vi "Build CHM.vi"() -> ()   [LabVIEW 2015]
uses:
  <vilib>/Utility/config.llb/Read Key (String).vi
  <vilib>/Utility/config.llb/Read Key (Path).vi
  Classes/CHM Generator/CHM Generator.lvclass
  <vilib>/Utility/config.llb/NI_LVConfig.lvlib
panel:
  out "standard output":string
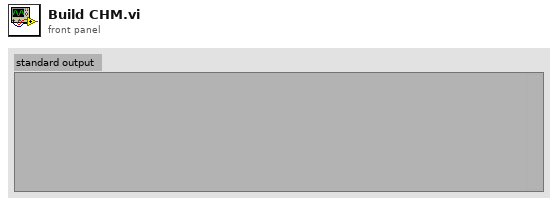
[diagram p1: front panel]
types:
  T1 = typedef "NI_LVConfig.lvlib/Config Data RefNum.ctl" = refnum<k1>
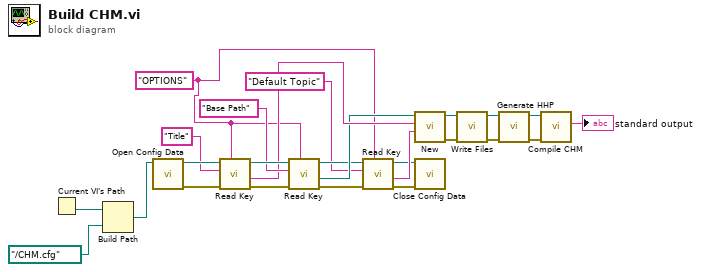
[diagram p0: block diagram]
diagram:
  w4 = "OPTIONS" ("section")
  n1 = Current VI's Path() -> (path=w3:path)
  n2 = Build Path(base path=w3, name or relative path=path "../CHM.cfg" ("Path")) -> (appended path=w1:path)
  n3 = call <vilib>:"Open Config Data.vi"("configuration file path"=w1) -> ("error out"=w17:errorcluster, "refnum"=w18:T1)  [unwired: 8 in, 1 out]
  n4 = call-poly <vilib>:"Read Key.vi"("section"=w4, "error in (no error)"=w17, "key"="Title", "refnum"=w18) -> ("error out"=w15:errorcluster, "value"=w12:string, "refnum out"=w14:T1)  [unwired: 4 in, 1 out]
  n5 = call-poly <vilib>:"Read Key.vi"("section"=w4, "error in (no error)"=w15, "key"="Base Path", "refnum"=w14) -> ("error out"=w11:errorcluster, "value"=w10:path, "refnum out"=w9:T1)  [unwired: 4 in, 1 out]
  n6 = call-poly <vilib>:"Read Key.vi"("section"=w4, "error in (no error)"=w11, "key"="Default Topic", "refnum"=w9) -> ("error out"=w6:errorcluster, "value"=w7:string, "refnum out"=w5:T1)  [unwired: 4 in, 1 out]
  n7 = call "New.vi"("Default topic"=w7, "Title"=w12, "Base Path"=w10) -> ("error out"=w24:errorcluster, "CHM Generator out"=w25:refnum<class "CHM Generator.lvclass">)  [unwired: 7 in]
  n8 = call <vilib>:"Close Config Data.vi"("error in (no error)"=w6, "refnum"=w5) -> ()  [unwired: 8 in, 2 out]
  n9 = call-dynamic "Write Files.vi"("error in (no error)"=w24, "CHM Generator in"=w25) -> ("error out"=w23:errorcluster, "CHM Generator out"=w22:refnum<class "CHM Generator.lvclass">)  [unwired: 8 in]
  n10 = call-dynamic "Generate HHP.vi"("error in (no error)"=w23, "CHM Generator in"=w22) -> ("error out"=w20:errorcluster, "CHM Generator out"=w21:refnum<class "CHM Generator.lvclass">)  [unwired: 8 in]
  n11 = call "Compile CHM.vi"("error in (no error)"=w20, "CHM Generator in"=w21) -> ("standard output"=→"standard output":string)  [unwired: 7 in, 2 out]
